vi "Analysis.Join CSV Data FIles.vi"(8 "OutputFile":path, 9 "InputFile2":path=path "C:/MTE/MTE Data Analysis/Reports/File2", 10 "InputFile1":path=path "C:/MTE/MTE Data Analysis/Reports/File1", 11 "Field to Join":string="SN") -> (0 "Error":errorcluster)   [LabVIEW 2024]
uses:
  Errors.lvlib
  <vilib>/KATE/Files/File Utils.lvlib
panel:
  in  "Stay Open":bool
  out "Active":bool
  in  "Cancel Button":bool
  in  "OK Button":bool
  in  "Join Type":T1(ring)
  in  "error in (no error)":errorcluster
  out "Data Out":string[][](table)
  # "Util - Join Tables in CSV Files"
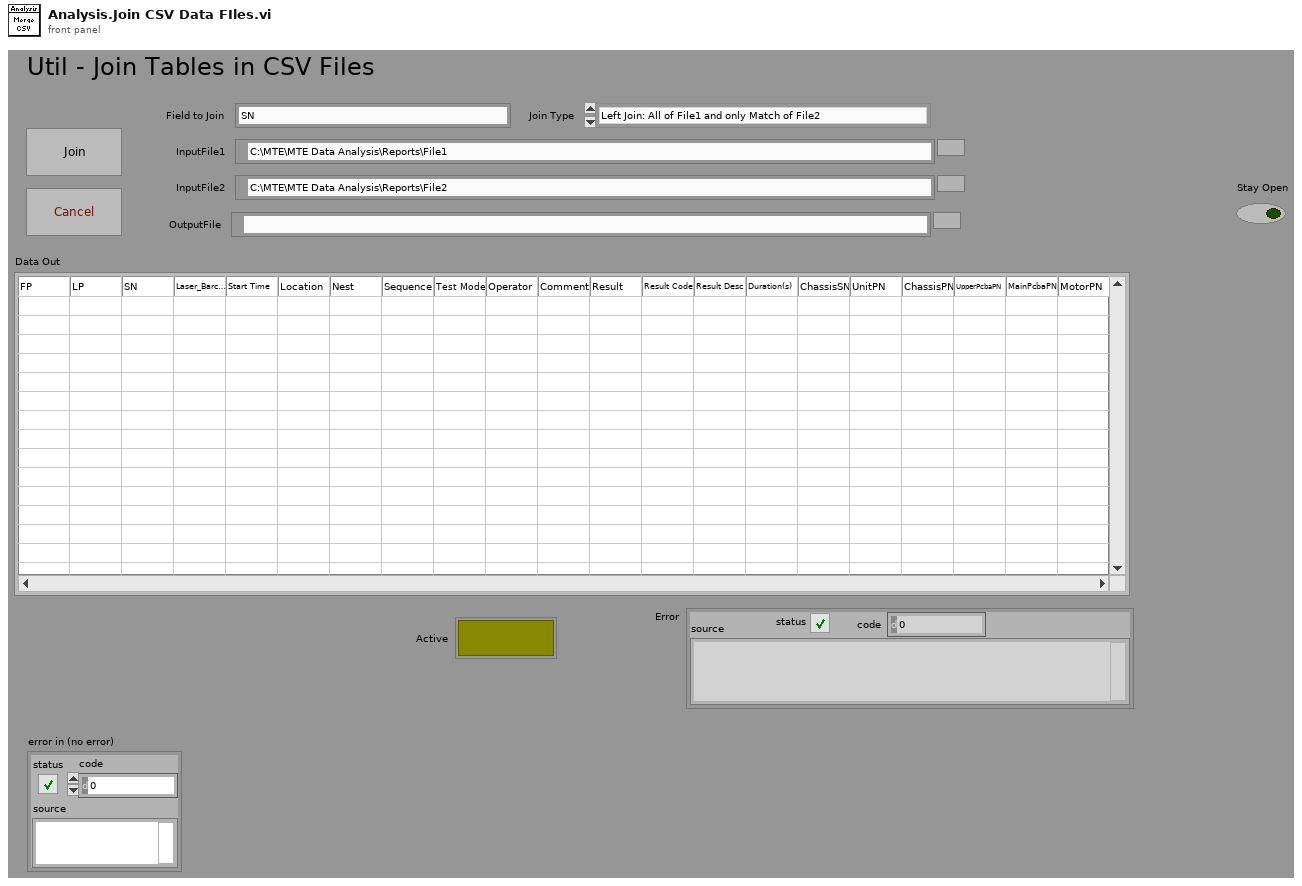
[diagram p1: front panel]
types:
  T1 = enum16{"Left Join: All of File1 and only Match of File2", "Right Join: All of File2 and only Match of File1"}
  T2 = cluster{"Header1":string[], "Data1":string[][], "Header2":string[], "Data2":string[][], "HeaderOut":string[], "DataOut":string[][], "JoinCol1":i32, "JoinCol2":i32, "Cancel":bool}
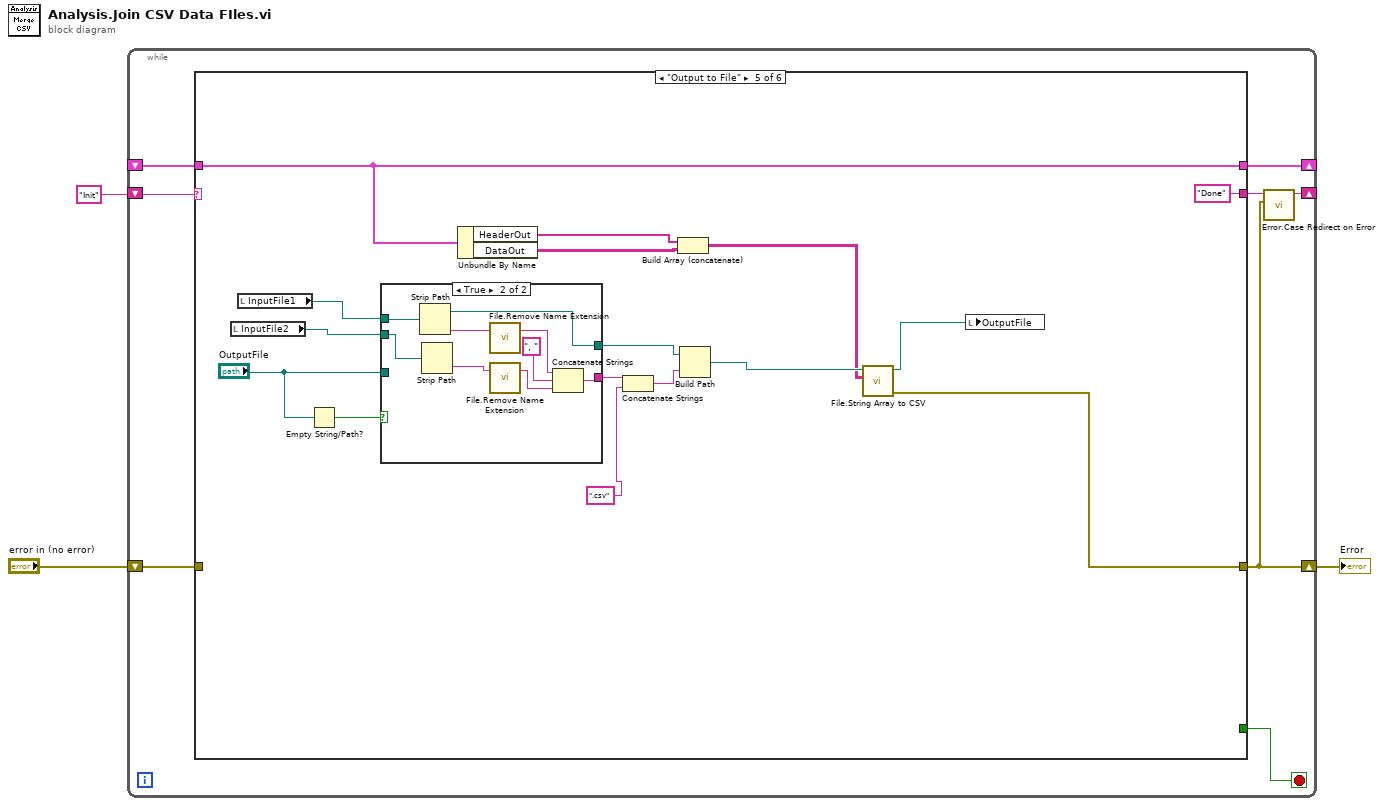
[diagram p0: block diagram]
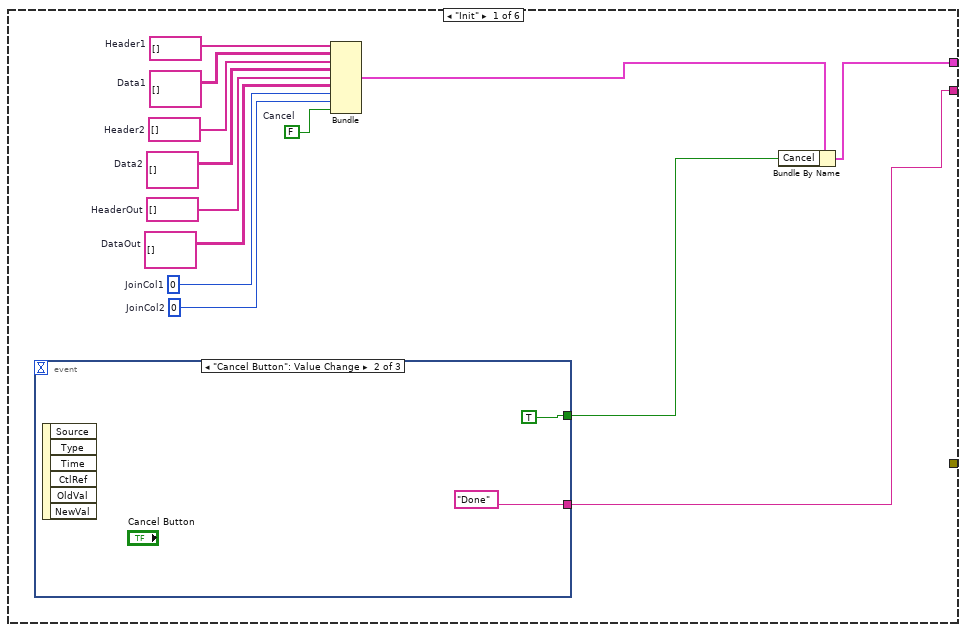
[diagram p2: hidden frame]
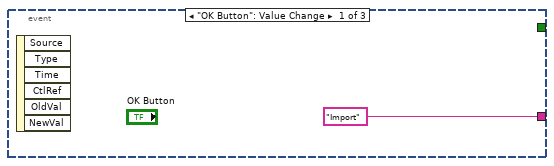
[diagram p3: hidden frame]
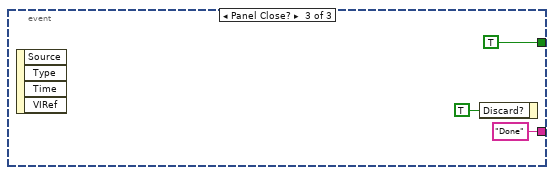
[diagram p4: hidden frame]
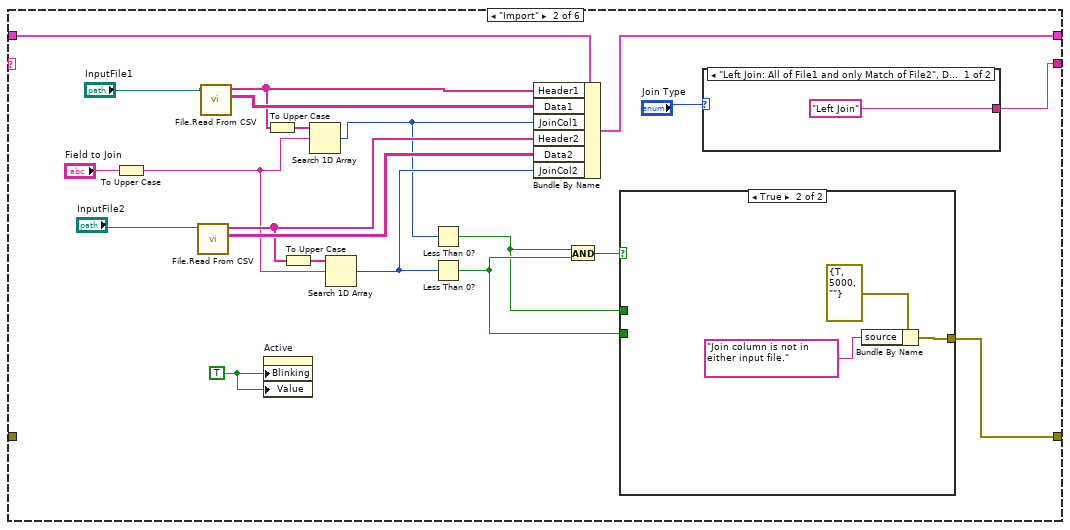
[diagram p5: hidden frame]
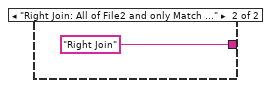
[diagram p6: hidden frame]
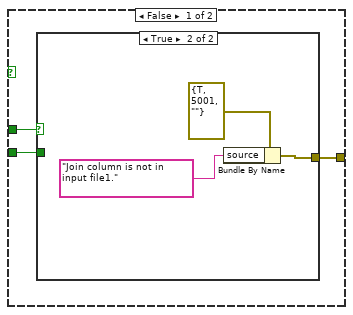
[diagram p7: hidden frame]
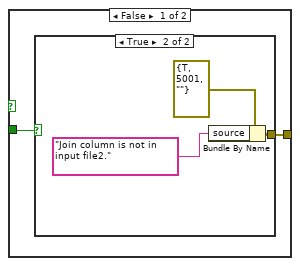
[diagram p8: hidden frame]
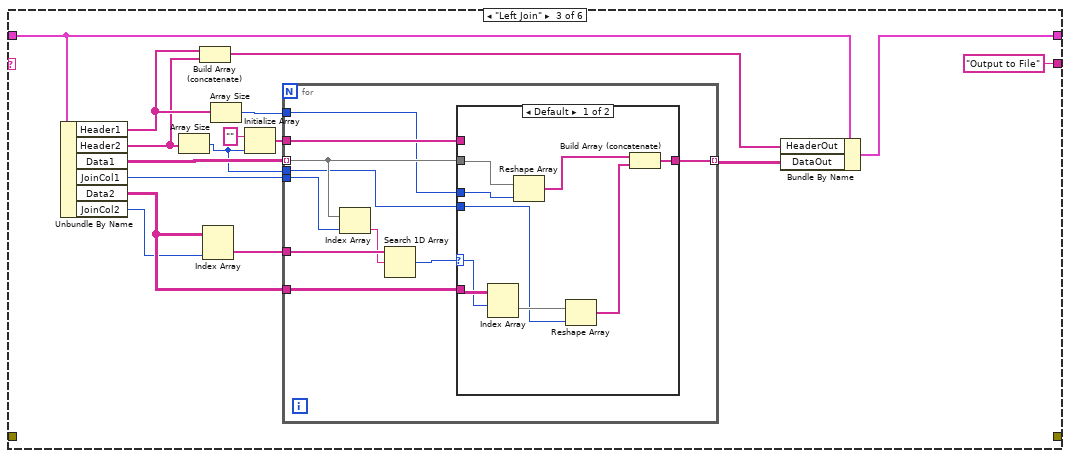
[diagram p10: hidden frame]
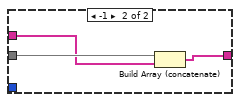
[diagram p11: hidden frame]
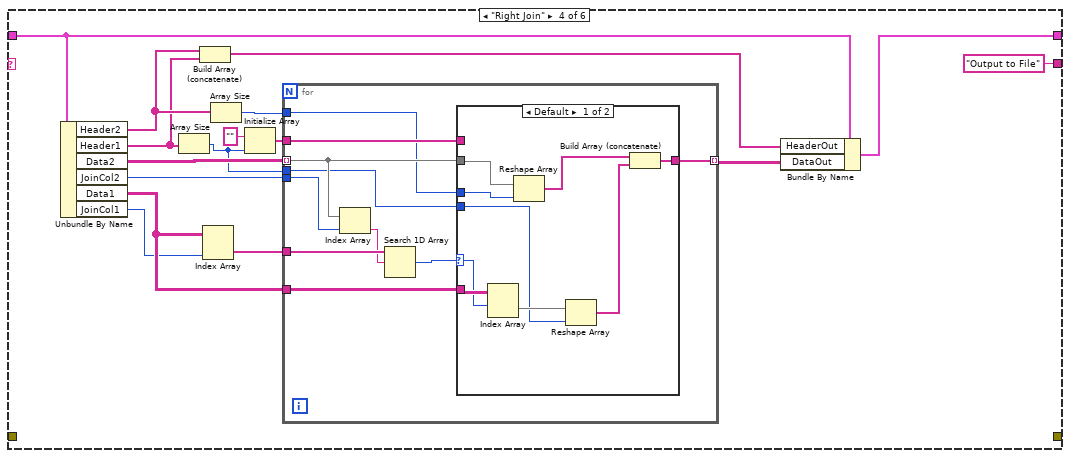
[diagram p12: hidden frame]
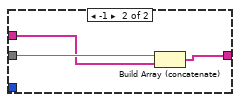
[diagram p13: hidden frame]
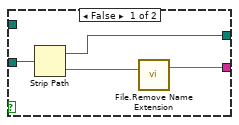
[diagram p14: hidden frame]
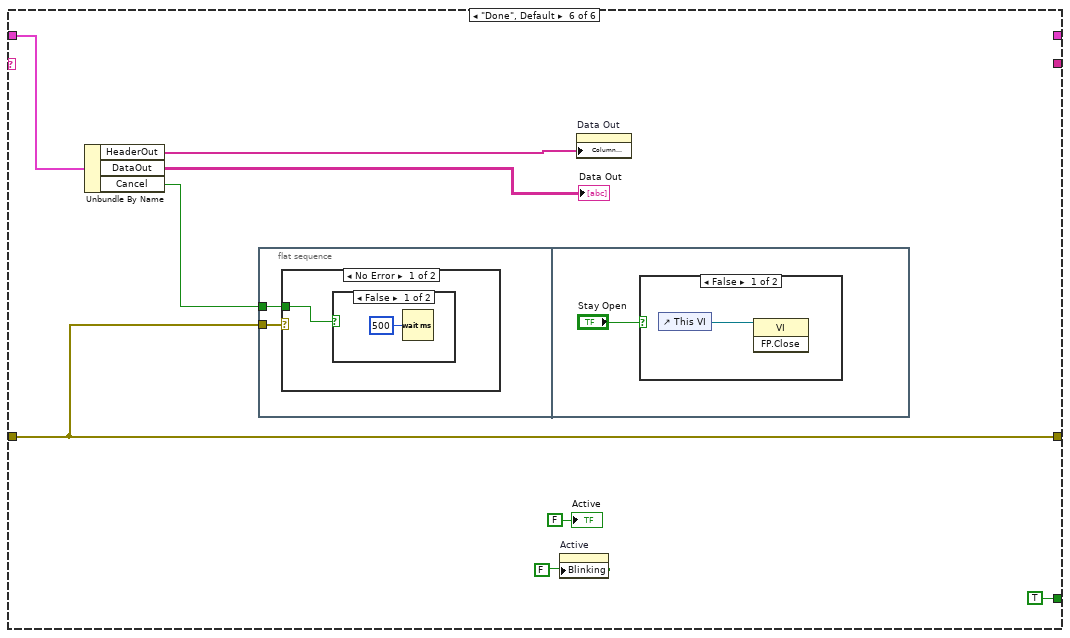
[diagram p15: hidden frame]
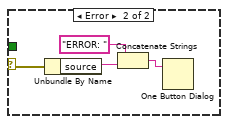
[diagram p17: hidden frame]
diagram:
  n1 = while {
    shift-right: [w5] -> w1
    shift-left: "error in (no error)" -> [w10]
    shift-right: [w7] -> _
    shift-left: "Init" -> [w11]
    shift-right: [w9] -> _
    shift-left: _ -> [w6]
    stop <- w4 stop-if-true
    n2 = case shown="\"Output to File\"" w11 {
      tunnel: w10 -> [_ _ _ _ _ w176]
      tunnel: [w13 w42 w75 w113 w158 _] -> w9
      tunnel: [w16 w34 "Output to File" "Output to File" "Done" _] -> w8
      tunnel: w6 -> [_ w51 w74 w112 w158 w179]
      tunnel: [_ w38 _ _ w147 w176] -> w5
      tunnel: [_ _ _ _ _ TRUE] -> w4
      frame "Init" {
        w15 = FALSE  # Cancel
        w17 = 0  # JoinCol2
        w18 = 0  # JoinCol1
        w19 = string[][] []  # DataOut
        w20 = string[] []  # HeaderOut
        w21 = string[][] []  # Data2
        w22 = string[] []  # Header2
        w23 = string[][] []  # Data1
        w24 = string[] []  # Header1
        n3 = event shown="[1] \"Cancel Button\": Value Change" {
          selector: _ -> [_ _ _]
          dyn-events: _ -> [_ _ _]
          timeout: _ -> [_ _ _]
          tunnel: ["Import" "Done" "Done"] -> w16
          tunnel: [_ TRUE TRUE] -> w12
          event "OK Button": Value Change {
            n4 = event-data() -> ()  [unwired: 1 in, 6 out]
          }
          event "Cancel Button": Value Change {
            n5 = event-data() -> ()  [unwired: 1 in, 6 out]
          }
          event Panel Close? {
            n6 = event-data() -> ()  [unwired: 1 in, 4 out]
            n7 = event-data("Discard?"=TRUE) -> ()  [unwired: 1 in, 1 out]
          }
        }
        n8 = Bundle("Header1"=w24, "Data1"=w23, "Header2"=w22, "Data2"=w21, "HeaderOut"=w20, "DataOut"=w19, "JoinCol1"=w18, "JoinCol2"=w17, "Cancel"=w15) -> (w14:T2)  [unwired: 1 in]
        n9 = Bundle By Name(cluster=w14, "Cancel"=w12) -> (w13:T2)
      }
      frame "Import" {
        w31 = TRUE ("Blinking")
        n10 = To Upper Case(1:"Field to Join") -> (0:w43:string)
        n11 = call <vilib>:"File.Read From CSV.vi"("File"="InputFile2") -> ("Data"=w49:string[][], "Header"=w47:string[])  [unwired: 8 in, 1 out]
        n12 = call <vilib>:"File.Read From CSV.vi"("File"="InputFile1") -> ("Data"=w50:string[][], "Header"=w44:string[])  [unwired: 8 in, 1 out]
        n13 = property on="Active" class="Bool (strict)"("Blinking"=w31, "Value"=w31) -> ()  [unwired: 2 in, 2 out]
        n14 = To Upper Case(1:w44) -> (0:w45:string[])
        n15 = To Upper Case(1:w47) -> (0:w46:string[])
        n16 = Search 1D Array(1D array=w45, element=w43) -> (index of element=w40:i32)  [unwired: 1 in]
        n17 = Search 1D Array(1D array=w46, element=w43) -> (index of element=w41:i32)  [unwired: 1 in]
        n18 = Less Than 0?(x=w40) -> (x < 0?=w36:bool)
        n19 = Less Than 0?(x=w41) -> (x < 0?=w37:bool)
        n20 = Bundle By Name(cluster=w51, "Header1"=w44, "Data1"=w50, "JoinCol1"=w40, "Header2"=w47, "Data2"=w49, "JoinCol2"=w41) -> (w42:T2)
        n21 = And(x=w36, y=w37) -> (x .and. y?=w39:bool)
        n22 = case shown="True" w39 {
          tunnel: [w54 w65] -> w38
          tunnel: w37 -> [w56 _]
          tunnel: w36 -> [w55 _]
          frame False {
            n23 = case shown="True" w55 {
              tunnel: w56 -> [w58 _]
              tunnel: [w57 w62] -> w54
              frame False {
                n24 = case shown="True" w58 {
                  tunnel: [_ w59] -> w57
                  frame False {
                  }
                  frame True {
                    n25 = Bundle By Name(cluster=errorcluster {"status"=TRUE, "code"=5001, "source"=""} ("error constant"), "source"="Join column is not in  input file2.") -> (w59:errorcluster)
                  }
                }
              }
              frame True {
                n26 = Bundle By Name(cluster=errorcluster {"status"=TRUE, "code"=5001, "source"=""} ("error constant"), "source"="Join column is not in  input file1.") -> (w62:errorcluster)
              }
            }
          }
          frame True {
            n27 = Bundle By Name(cluster=errorcluster {"status"=TRUE, "code"=5000, "source"=""} ("error constant"), "source"="Join column is not in either input file.") -> (w65:errorcluster)
          }
        }
        n28 = case shown="\"Left Join: All of File1 and only Match of File2\", Default" "Join Type" {
          tunnel: ["Left Join" "Right Join"] -> w34
          frame "Left Join: All of File1 and only Match of File2", Default {
          }
          frame "Right Join: All of File2 and only Match of File1" {
          }
        }
      }
      frame "Left Join" {
        n29 = Unbundle By Name(w74) -> ("Header1"=w73:string[], "Header2"=w72:string[], "Data1"=w82:string[][], "JoinCol1"=w81:i32, "Data2"=w80:string[][], "JoinCol2"=w79:i32)
        n30 = Array Size(array=w72) -> (size(s)=w68:i32)
        n31 = Build Array (concatenate)(w73, w72) -> (w76:string[])
        n32 = Index Array(array=w80, index (col)=w79) -> (element=w78:string[])  [unwired: 1 in]
        n33 = Array Size(array=w73) -> (size(s)=w71:i32)
        n34 = Initialize Array("", w68) -> (w69:string[])
        n35 = for {
          tunnel: w82 -> [w89] mode=indexing
          tunnel: w81 -> [w93]
          tunnel: w80 -> [w87]
          tunnel: w78 -> [w92]
          tunnel: [w88] -> w77 mode=indexing
          tunnel: w71 -> [w85]
          tunnel: w69 -> [w86]
          tunnel: w68 -> [w84]
          n36 = Index Array(array=w89, index=w93) -> (element=w91:string)
          n37 = Search 1D Array(1D array=w92, element=w91) -> (index of element=w90:i32)  [unwired: 1 in]
          n38 = case shown="Default" w90 {
            selector: w90 -> [w101 _]
            tunnel: w89 -> [w98 w105]
            tunnel: [w100 w104] -> w88
            tunnel: w87 -> [w102 _]
            tunnel: w86 -> [_ w103]
            tunnel: w85 -> [w99 _]
            tunnel: w84 -> [w94 _]
            frame Default {
              n39 = Index Array(array=w102, index (row)=w101) -> (element=w96:string[])  [unwired: 1 in]
              n40 = Reshape Array(w98, w99) -> (w97:string[])
              n41 = Reshape Array(w96, w94) -> (w95:string[])
              n42 = Build Array (concatenate)(w97, w95) -> (w100:string[])
            }
            frame -1 {
              n43 = Build Array (concatenate)(w105, w103) -> (w104:string[])
            }
          }
        }
        n44 = Bundle By Name(cluster=w74, "HeaderOut"=w76, "DataOut"=w77) -> (w75:T2)
      }
      frame "Right Join" {
        n45 = Unbundle By Name(w112) -> ("Header2"=w111:string[], "Header1"=w110:string[], "Data2"=w120:string[][], "JoinCol2"=w119:i32, "Data1"=w118:string[][], "JoinCol1"=w117:i32)
        n46 = Array Size(array=w110) -> (size(s)=w106:i32)
        n47 = Build Array (concatenate)(w111, w110) -> (w114:string[])
        n48 = Index Array(array=w118, index (col)=w117) -> (element=w116:string[])  [unwired: 1 in]
        n49 = Array Size(array=w111) -> (size(s)=w109:i32)
        n50 = Initialize Array("", w106) -> (w107:string[])
        n51 = for {
          tunnel: w120 -> [w127] mode=indexing
          tunnel: w119 -> [w131]
          tunnel: w118 -> [w125]
          tunnel: w116 -> [w130]
          tunnel: [w126] -> w115 mode=indexing
          tunnel: w109 -> [w123]
          tunnel: w107 -> [w124]
          tunnel: w106 -> [w122]
          n52 = Index Array(array=w127, index=w131) -> (element=w129:string)
          n53 = Search 1D Array(1D array=w130, element=w129) -> (index of element=w128:i32)  [unwired: 1 in]
          n54 = case shown="Default" w128 {
            selector: w128 -> [w139 _]
            tunnel: w127 -> [w136 w143]
            tunnel: [w138 w142] -> w126
            tunnel: w125 -> [w140 _]
            tunnel: w124 -> [_ w141]
            tunnel: w123 -> [w137 _]
            tunnel: w122 -> [w132 _]
            frame Default {
              n55 = Index Array(array=w140, index (row)=w139) -> (element=w134:string[])  [unwired: 1 in]
              n56 = Reshape Array(w136, w137) -> (w135:string[])
              n57 = Reshape Array(w134, w132) -> (w133:string[])
              n58 = Build Array (concatenate)(w135, w133) -> (w138:string[])
            }
            frame -1 {
              n59 = Build Array (concatenate)(w143, w141) -> (w142:string[])
            }
          }
        }
        n60 = Bundle By Name(cluster=w112, "HeaderOut"=w114, "DataOut"=w115) -> (w113:T2)
      }
      frame "Output to File" {
        n61 = local read "InputFile2"() -> (w154:path)
        n62 = local read "InputFile1"() -> (w155:path)
        n63 = Empty String/Path?(string/path="OutputFile") -> (empty?=w157:bool)
        n64 = case shown="True" w157 {
          tunnel: w155 -> [_ w172]
          tunnel: w154 -> [_ w171]
          tunnel: "OutputFile" -> [w163 _]
          tunnel: [w161 w167] -> w153
          tunnel: [w160 w168] -> w150
          frame False {
            n65 = Strip Path(path=w163) -> (stripped path=w160:path, name=w162:string)
            n66 = call <vilib>:"File.Remove Name Extension.vi"("File Name"=w162) -> ("Name Less Ext"=w161:string)  [unwired: 1 in, 1 out]
          }
          frame True {
            n67 = Strip Path(path=w172) -> (stripped path=w168:path, name=w169:string)
            n68 = Strip Path(path=w171) -> (name=w170:string)  [unwired: 1 out]
            n69 = call <vilib>:"File.Remove Name Extension.vi"("File Name"=w169) -> ("Name Less Ext"=w166:string)  [unwired: 1 in, 1 out]
            n70 = call <vilib>:"File.Remove Name Extension.vi"("File Name"=w170) -> ("Name Less Ext"=w164:string)  [unwired: 1 in, 1 out]
            n71 = Concatenate Strings(w166, ", ", w164) -> (w167:string)
          }
        }
        n72 = Unbundle By Name(w158) -> ("HeaderOut"=w146:string[], "DataOut"=w145:string[][])
        n73 = Concatenate Strings(w153, ".csv") -> (w151:string)
        n74 = Build Array (concatenate)(w146, w145) -> (w144:string[][])
        n75 = Build Path(base path=w150, name or relative path=w151) -> (appended path=w149:path)
        n76 = call "File.String Array to CSV.vi"("2D Str"=w144, "FilePath"=w149) -> ("Error Out"=w147:errorcluster, "FilePath Out"=w148:path)  [unwired: 8 in]
        n77 = local write "OutputFile"(w148) -> ()
      }
      frame "Done", Default {
        n78 = Unbundle By Name(w179) -> ("HeaderOut"=w177:string[], "DataOut"=→"Data Out":string[][], "Cancel"=w175:bool)
        n79 = flat-sequence {
          tunnel: w176 -> [w182]
          tunnel: w175 -> [w181]
          frame #0 {
            n80 = case shown="No Error" w182 {
              selector: w182 -> [_ w188]
              tunnel: w181 -> [w183 _]
              frame No Error {
                n81 = case shown="False" w183 {
                  frame False {
                    n82 = Wait (ms)(milliseconds to wait=u32 500) -> ()  [unwired: 1 out]
                  }
                  frame True {
                  }
                }
              }
              frame Error {
                n83 = Unbundle By Name(w188) -> ("source"=w186:string)
                n84 = Concatenate Strings("ERROR: ", w186) -> (w185:string)
                n85 = One Button Dialog(message=w185) -> ()  [unwired: 1 in, 1 out]
              }
            }
          }
          frame #1 {
            n86 = case shown="False" "Stay Open" {
              frame False {
                n87 = control-ref of="This VI"() -> (w190:refnum<vi>)
                n88 = invoke class="VI" method="FP.Close"(reference=w190) -> ()  [unwired: 2 in, 3 out]
              }
              frame True {
              }
            }
          }
        }
        n89 = property on="Active" class="Bool (strict)"("Blinking"=FALSE) -> ()  [unwired: 2 in, 2 out]
        n90 = property on="Data Out" class="Tbl (strict)"("Column Headers[]"=w177) -> ()  [unwired: 2 in, 2 out]
        "Active" <- FALSE ("Active")
      }
    }
    n91 = call "Error.Case Redirect on Error.vi"("error in"=w5, "Next Case"=w8) -> ("Next Case Out"=w7:string)  [unwired: 9 in]
  }
  "Error" <- w1
